vi "Read File Header.vi"(0 "reference in":refnum<class "RPC.lvclass">, 5 "error in (no error)":errorcluster) -> (14 "reference out":refnum<class "RPC.lvclass">, 19 "error out":errorcluster)   [LabVIEW 2022 SP3, in "RPC.lvclass"]
uses:
  RPC.lvclass
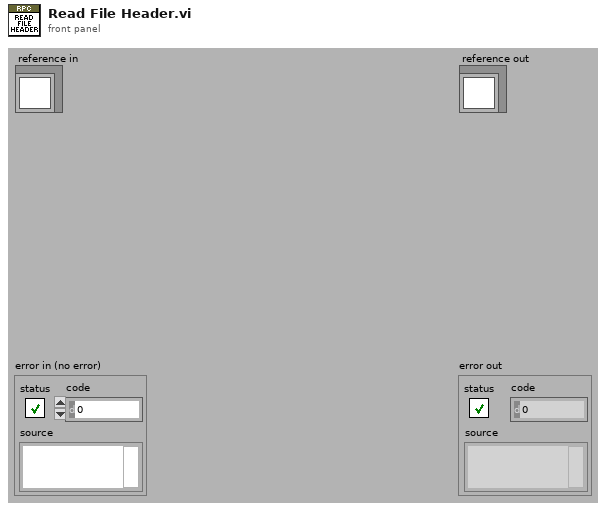
[diagram p1: front panel]
types:
  T1 = typedef "RPC.lvclass/ObjectAttributesRef.ctl" = refnum<data-value>
  T2 = typedef "RPC.lvclass/ObjectAttributes.ctl" = cluster{"File Refnum":refnum<file>, "File total size":i32, "Offset from start of file":i32, "Time Type":enum16{"Response", "Drive"}, "Full Scale":dbl[unit], "New Time Data Obj?":bool, "Header":cluster{"Num Header":i32, "Num Parameter":i32, "Nb Channels":i32, "dT":dbl, "Number of Groups":i32, "Group size":i32, "Units":string[], "Names":string[], "Sensitivity":dbl[], "Complete header":string[]}, "Time Data":refnum<class "GSwFormDSP.lvclass">}
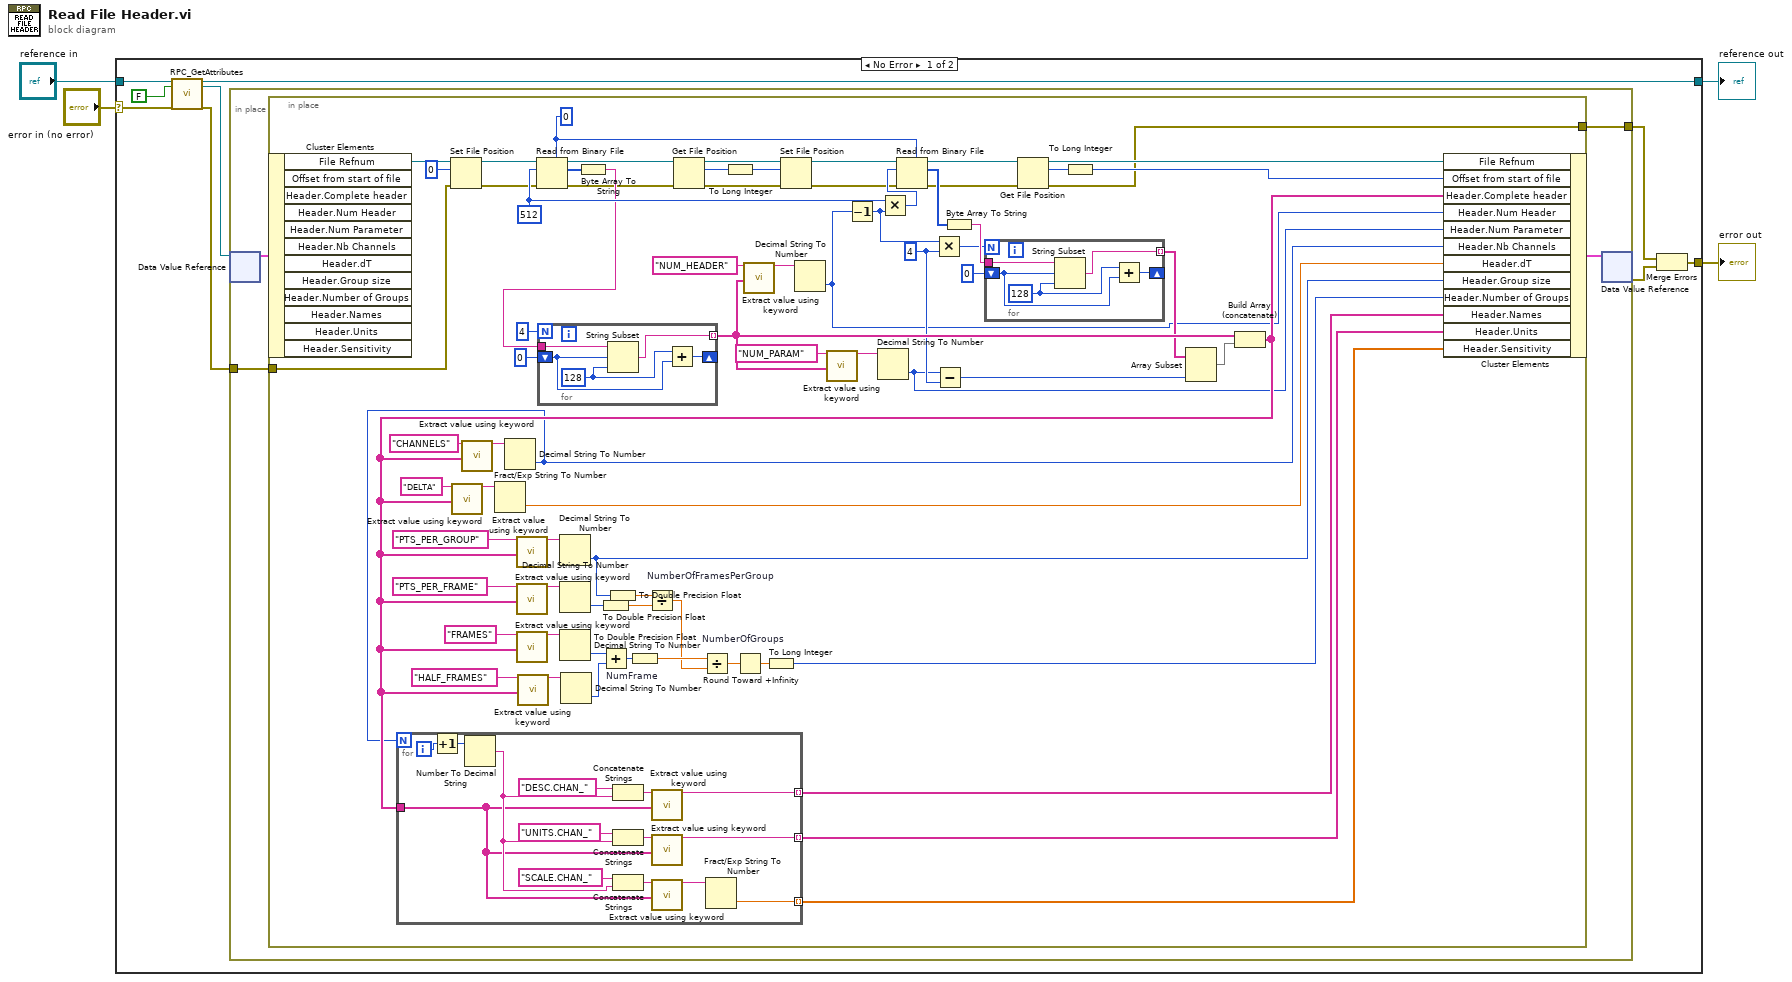
[diagram p0: block diagram]
diagram:
  n1 = case shown="No Error" "error in (no error)" {
    selector: "error in (no error)" -> [w9 w115]
    tunnel: [w13 w115] -> w3
    tunnel: [w8 w114] -> w1
    tunnel: "reference in" -> [w11 w114]
    frame No Error {
      n2 = call "RPC_GetAttributes.vi"("reference in"=w11, "return data? (T)"=FALSE, "error in (no error)"=w9) -> ("reference out"=w8:refnum<class "RPC.lvclass">, "attributes ref"=w7:T1, "error out"=w6:errorcluster)  [unwired: 13 in, 1 out]
      n3 = in-place {
        in-place-border: w6 -> [w15]
        in-place-border: [w14] -> w5
        n4 = in-place-dvr #1(w7) -> (w16:T2)  [unwired: 1 out]
        n5 = in-place {
          in-place-border: w15 -> [w32]
          in-place-border: [w18] -> w14
          w68 = 4
          w89 = u8 0
          w83 = 512 ("count")
          n6 = in-place-cluster #2(w16) -> ("File Refnum"=w31:refnum<file>)  [unwired: 11 out]
          n7 = Set File Position(offset (in bytes) (0)=0 ("pos offset (0)"), refnum=w31, error in=w32) -> (refnum out=w37:refnum<file>, error out=w36:errorcluster)  [unwired: 1 out]
          n8 = Read from Binary File(5:w89, 8:w36, 10:w83, 11:w37) -> (0:w34:errorcluster, 2:w88:u8[], 3:w35:refnum<file>)  [unwired: 3 out]
          n9 = Byte Array To String(unsigned byte array=w88) -> (string=w79:string)
          n10 = for {
            N: 4 -> [_]
            tunnel: w79 -> [w113]
            shift-right: [w110] -> _
            shift-left: 0 -> [w111]
            tunnel: [w109] -> w69 mode=indexing
            w112 = 128 ("length (rest)")
            n11 = String Subset(string=w113, offset (0)=w111, length (rest)=w112) -> (substring=w109:string)
            n12 = Add(x=w112, y=w111) -> (x+y=w110:i32)
          }
          n13 = Get File Position(4:w34, 7:w35) -> (0:w84:errorcluster, 2:w33:i64, 3:w86:refnum<file>)
          n14 = To Long Integer(number=w33) -> (32bit integer=w85:i32)
          n15 = call "Extract value using keyword.vi"("Keyword"="NUM_HEADER", "Header"=w69) -> ("Value"=w76:string)  [unwired: 17 in]
          n16 = Set File Position(offset (in bytes) (0)=w85, refnum=w86, error in=w84) -> (refnum out=w42:refnum<file>, error out=w41:errorcluster)  [unwired: 1 out]
          n17 = Decimal String To Number(string=w76) -> (number=w27:i32)  [unwired: 3 out]
          n18 = call "Extract value using keyword.vi"("Keyword"="NUM_PARAM", "Header"=w69) -> ("Value"=w71:string)  [unwired: 17 in]
          n19 = Decrement(x=w27) -> (x-1=w73:i32)
          n20 = Decimal String To Number(string=w71) -> (number=w26:i32)  [unwired: 3 out]
          n21 = Multiply(x=w83, y=w73) -> (x*y=w82:i32)
          n22 = Read from Binary File(5:w89, 8:w41, 10:w82, 11:w42) -> (0:w39:errorcluster, 2:w81:u8[], 3:w40:refnum<file>)  [unwired: 3 out]
          n23 = Multiply(x=w73, y=w68) -> (x*y=w72:i32)
          n24 = Subtract(x=w26, y=w68) -> (x-y=w66:i32)
          n25 = Byte Array To String(unsigned byte array=w81) -> (string=w74:string)
          n26 = for {
            N: w72 -> [_]
            tunnel: w74 -> [w108]
            shift-right: [w105] -> _
            shift-left: 0 -> [w106]
            tunnel: [w104] -> w67 mode=indexing
            w107 = 128 ("length (rest)")
            n27 = String Subset(string=w108, offset (0)=w106, length (rest)=w107) -> (substring=w104:string)
            n28 = Add(x=w107, y=w106) -> (x+y=w105:i32)
          }
          n29 = Get File Position(4:w39, 7:w40) -> (0:w18:errorcluster, 2:w38:i64, 3:w30:refnum<file>)
          n30 = To Long Integer(number=w38) -> (32bit integer=w29:i32)
          n31 = Array Subset(array=w67, length=w66) -> (w65:string[])  [unwired: 1 in]
          n32 = Build Array (concatenate)(w69, w65) -> (w28:string[])
          n33 = call "Extract value using keyword.vi"("Keyword"="DELTA", "Header"=w28) -> ("Value"=w62:string)  [unwired: 17 in]
          n34 = call "Extract value using keyword.vi"("Keyword"="CHANNELS", "Header"=w28) -> ("Value"=w63:string)  [unwired: 17 in]
          n35 = Fract/Exp String To Number(string=w62) -> (number=w24:dbl)  [unwired: 4 out]
          n36 = Decimal String To Number(string=w63) -> (number=w25:i32)  [unwired: 3 out]
          n37 = for {
            N: w25 -> [_]
            tunnel: w28 -> [w92]
            tunnel: [w99] -> w21 mode=indexing
            tunnel: [w96] -> w20 mode=indexing
            tunnel: [w90] -> w19 mode=indexing
            i -> [w103]
            n38 = Increment(x=w103) -> (x+1=w102:i32)
            n39 = Number To Decimal String(number=w102) -> (decimal integer string=w93:string)  [unwired: 1 out]
            n40 = Concatenate Strings("DESC.CHAN_", w93) -> (w100:string)
            n41 = Concatenate Strings("UNITS.CHAN_", w93) -> (w98:string)
            n42 = Concatenate Strings("SCALE.CHAN_", w93) -> (w94:string)
            n43 = call "Extract value using keyword.vi"("Keyword"=w100, "Header"=w92) -> ("Value"=w99:string)  [unwired: 17 in]
            n44 = call "Extract value using keyword.vi"("Keyword"=w98, "Header"=w92) -> ("Value"=w96:string)  [unwired: 17 in]
            n45 = call "Extract value using keyword.vi"("Keyword"=w94, "Header"=w92) -> ("Value"=w91:string)  [unwired: 17 in]
            n46 = Fract/Exp String To Number(string=w91) -> (number=w90:dbl)  [unwired: 4 out]
          }
          n47 = call "Extract value using keyword.vi"("Keyword"="PTS_PER_GROUP", "Header"=w28) -> ("Value"=w60:string)  [unwired: 17 in]
          n48 = call "Extract value using keyword.vi"("Keyword"="PTS_PER_FRAME", "Header"=w28) -> ("Value"=w57:string)  [unwired: 17 in]
          n49 = call "Extract value using keyword.vi"("Keyword"="FRAMES", "Header"=w28) -> ("Value"=w53:string)  [unwired: 17 in]
          n50 = call "Extract value using keyword.vi"("Keyword"="HALF_FRAMES", "Header"=w28) -> ("Value"=w50:string)  [unwired: 17 in]
          n51 = Decimal String To Number(string=w60) -> (number=w23:i32)  [unwired: 3 out]
          n52 = Decimal String To Number(string=w57) -> (number=w56:i32)  [unwired: 3 out]
          n53 = Decimal String To Number(string=w53) -> (number=w49:i32)  [unwired: 3 out]
          n54 = Decimal String To Number(string=w50) -> (number=w48:i32)  [unwired: 3 out]
          n55 = To Double Precision Float(number=w56) -> (double precision float=w54:dbl)
          n56 = Add "NumFrame"(x=w49, y=w48) -> (x+y=w46:i32)
          n57 = To Double Precision Float(number=w23) -> (double precision float=w55:dbl)
          n58 = To Double Precision Float(number=w46) -> (double precision float=w47:dbl)
          n59 = Divide "NumberOfFramesPerGroup"(x=w55, y=w54) -> (x/y=w45:dbl)
          n60 = Divide "NumberOfGroups"(x=w47, y=w45) -> (x/y=w44:dbl)
          n61 = Round Toward +Infinity(x=w44) -> (ceil(x): smallest int >= x=w43:dbl)
          n62 = To Long Integer(number=w43) -> (32bit integer=w22:i32)
          n63 = in-place-cluster #2("File Refnum"=w30, "Offset from start of file"=w29, "Header.Complete header"=w28, "Header.Num Header"=w27, "Header.Num Parameter"=w26, "Header.Nb Channels"=w25, "Header.dT"=w24, "Header.Group size"=w23, "Header.Number of Groups"=w22, "Header.Names"=w21, "Header.Units"=w20, "Header.Sensitivity"=w19) -> (w17:T2)
        }
        n64 = in-place-dvr #1(w17) -> (w12:errorcluster)  [unwired: 1 out]
      }
      n65 = Merge Errors(w5, w12) -> (w13:errorcluster)
    }
    frame Error {
    }
  }
  "error out" <- w3
  "reference out" <- w1
